vi "单点权值.vi"(0 "当前棋盘状态":i32[][](array[numeric]), 5 "黑棋棋盘权值初始":sgl[][](array[numeric]), 7 "行":sgl, 9 "列":i16, 11 "白棋棋盘权值初始":sgl[][](array[numeric])) -> (4 "当前棋盘状态":i32[][](array[numeric]), 6 "黑子棋盘权值":sgl[][](array[numeric]), 8 "白子棋盘权值":sgl[][](array[numeric]))   [LabVIEW 2018]
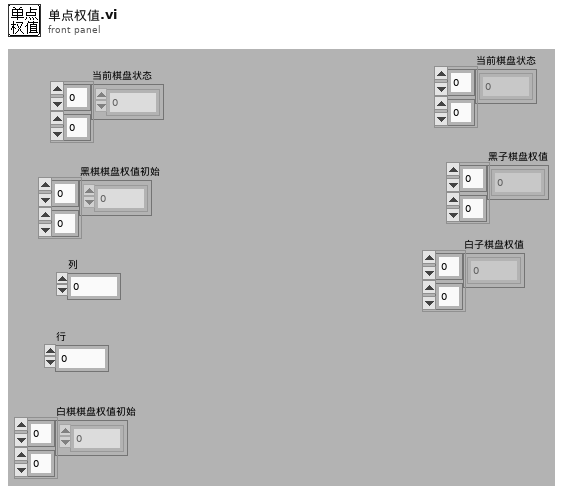
[diagram p1: front panel]
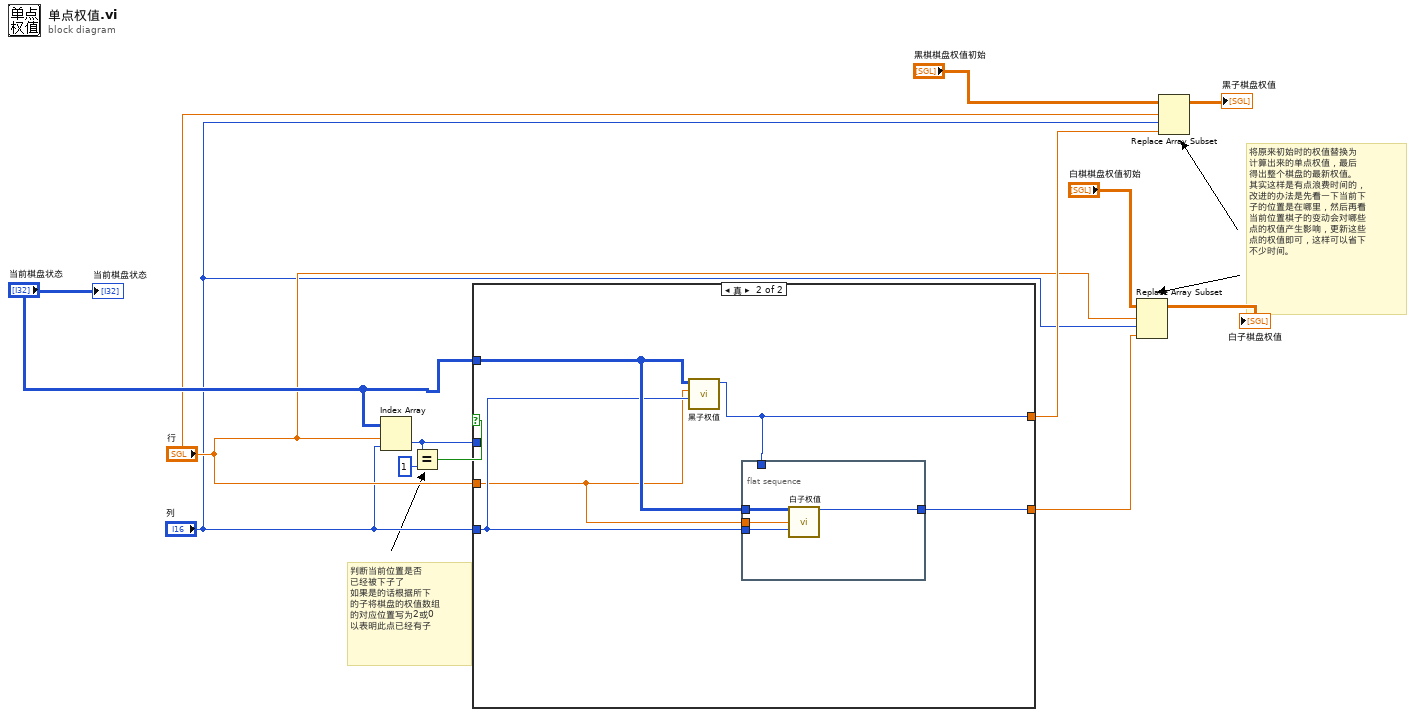
[diagram p0: block diagram]
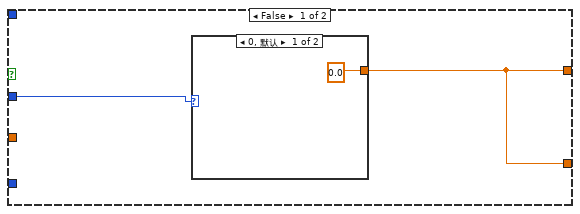
[diagram p2: hidden frame]
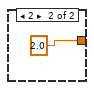
[diagram p3: hidden frame]
diagram:
  # "判断当前位置是否\n已经被下子了\n如果是的话根据所下\n的子将棋盘的权值数组\n的对应位置写为2或0\n以表明此点已经有子"
  # "将原来初始时的权值替换为\n计算出来的单点权值，最后\n得出整个棋盘的最新权值。\n其实这样是有点浪费时间的，\n改进的办法是先看一下当前下\n子的位置是在哪里，然后再看\n当前位置棋子的变动会对哪些\n点的权值产生影响，更新这些\n点的权值即可，这样可以省下\n不少时间。"
  n1 = Index Array(array="当前棋盘状态", index (row)="行", index (col)="列") -> (element=w1:i32)
  n2 = Equal?(x=w1, y=1) -> (x = y?=w8:bool)
  n3 = case shown="真" w8 {
    tunnel: "当前棋盘状态" -> [_ w21]
    tunnel: "列" -> [_ w20]
    tunnel: "行" -> [_ w18]
    tunnel: [w13 w17] -> w10
    tunnel: [w13 w19] -> w6
    tunnel: w1 -> [w14 _]
    frame False {
      n4 = case shown="0, 默认" w14 {
        tunnel: [sgl 0.0 sgl 2.0] -> w13
        frame 0, Default {
        }
        frame 2 {
        }
      }
    }
    frame True {
      n5 = call "黑子权值.vi"("列"=w20, "行"=w18, "当前棋盘状态"=w21) -> ("黑子总权值"=w17:i32)  [unwired: 8 in]
      n6 = flat-sequence {
        tunnel: w21 -> [w25]
        tunnel: w20 -> [w24]
        tunnel: [w23] -> w19
        tunnel: w18 -> [w22]
        tunnel: w17 -> [_]
        frame #0 {
          n7 = call "白子权值.vi"("当前棋盘状态"=w25, "行"=w22, "列"=w24) -> ("白子总权值"=w23:i32)  [unwired: 12 in]
        }
      }
    }
  }
  n8 = Replace Array Subset(array="白棋棋盘权值初始", new element=w6, index (row)="行", index (col)="列") -> (→"白子棋盘权值":sgl[][])
  n9 = Replace Array Subset(array="黑棋棋盘权值初始", new element=w10, index (row)="行", index (col)="列") -> (→"黑子棋盘权值":sgl[][])
  "当前棋盘状态" <- "当前棋盘状态"
